vi "Edit Operations.vi"(8 "error in (no error)":errorcluster caption="entrée d'erreur (pas d'erreur)", 9 "Parameters":T1, 10 "Key":i32, 11 "Operations en entrée":refnum<class "Operations.lvclass"> caption="DNL_LabVIEW Object in") -> (0 "error out":errorcluster caption="sortie d'erreur", 1 "created new?":bool, 3 "Operations en sortie":refnum<class "Operations.lvclass"> caption="DNL_LabVIEW Object out")   [LabVIEW 2012, in "Operations.lvclass"]
uses:
  Operations.lvclass
  Operation/Operation Parameters.ctl
  Operation/Operation Type Enum.ctl
  controls/Currencies.ctl
  <userlib>/_OpenG.lib/dictionary/dictionary.llb/Dictionary Key Value Pair Cluster__ogtk.ctl
  Operations.lvclass/Operations.ctl
  <userlib>/_OpenG.lib/dictionary/dictionary.llb/Dictionary Update (by scalar value)__ogtk.vi
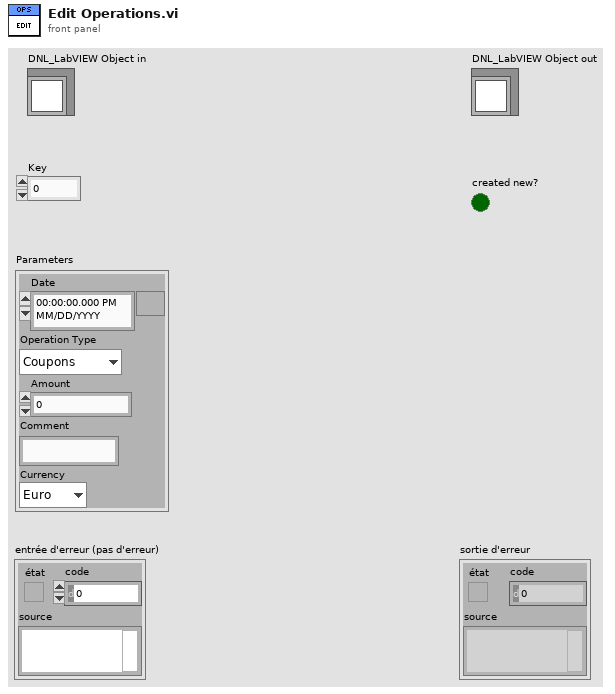
[diagram p1: front panel]
types:
  T1 = typedef "Operation Parameters.ctl" = cluster{"Date":timestamp, "Operation Type":T2, "Amount":dbl, "Comment":string, "Currency":T3}
  T2 = typedef "Operation Type Enum.ctl" = enum16{"Coupons", "Dépot", "Retrait", "Intérêts", "Taxe"}
  T3 = typedef "Currencies.ctl" = enum16{"Euro", "Dollar", "Yen", "RIM", "CHF"}
  T4 = typedef "Dictionary Key Value Pair Cluster__ogtk.ctl" = cluster{"key":variant, "value":variant}
  T5 = typedef "Dictionary Object RefNum__ogtk.ctl" = refnum<k1>
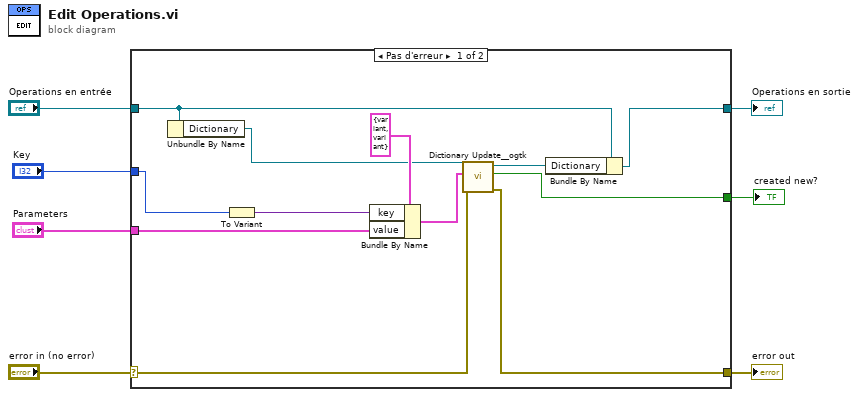
[diagram p0: block diagram]
diagram:
  n1 = case shown="Pas d'erreur" "error in (no error)" {
    selector: "error in (no error)" -> [w10 w21]
    tunnel: [w16 w21] -> w6
    tunnel: [w18 w20] -> w4
    tunnel: "Operations en entrée" -> [w19 w20]
    tunnel: [w15 _] -> w3
    tunnel: "Parameters" -> [w12 _]
    tunnel: "Key" -> [w9 _]
    frame No Error {
      n2 = Unbundle By Name(w19) -> ("Dictionary"=w11:T5)
      n3 = To Variant(anything=w9) -> (Variant=w8:variant)
      n4 = Bundle By Name(cluster=T4 {"key"=variant, "value"=variant} ("key-value"), "key"=w8, "value"=w12) -> (w13:T4)
      n5 = call-poly <userlib>:"Dictionary Update__ogtk.vi"("error in (no error)"=w10, "key-value"=w13, "dictionary"=w11) -> ("error out"=w16:errorcluster, "created new?"=w15:bool, "dictionary out"=w17:T5)  [unwired: 6 in]
      n6 = Bundle By Name(cluster=w19, "Dictionary"=w17) -> (w18:refnum<class "Operations.lvclass">)
    }
    frame Error {
    }
  }
  "error out" <- w6
  "Operations en sortie" <- w4
  "created new?" <- w3
